vi "ProFile_Measure.vi"(1 "Ceiling":sgl=4.0, 2 "error in":errorcluster caption="Error In") -> (0 "error out":errorcluster caption="Error Out")   [LabVIEW 2016]
doc: "2D motor scan example Vi."
uses:
  Utility/Global Constants.vi
  Utility/Global_Array.vi
  Utility/Global_Stage.vi
panel:
  in  "Y-Axis Scanner align":sgl=0.15
  in  "X-Axis Scanner align":sgl=-0.64
  out "Value Handle":dbl[](array[numeric])
  out "Status?":bool
  out "RS":bool
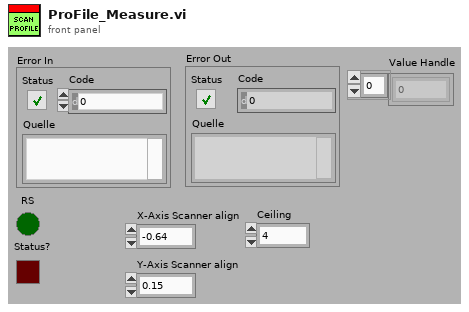
[diagram p1: front panel]
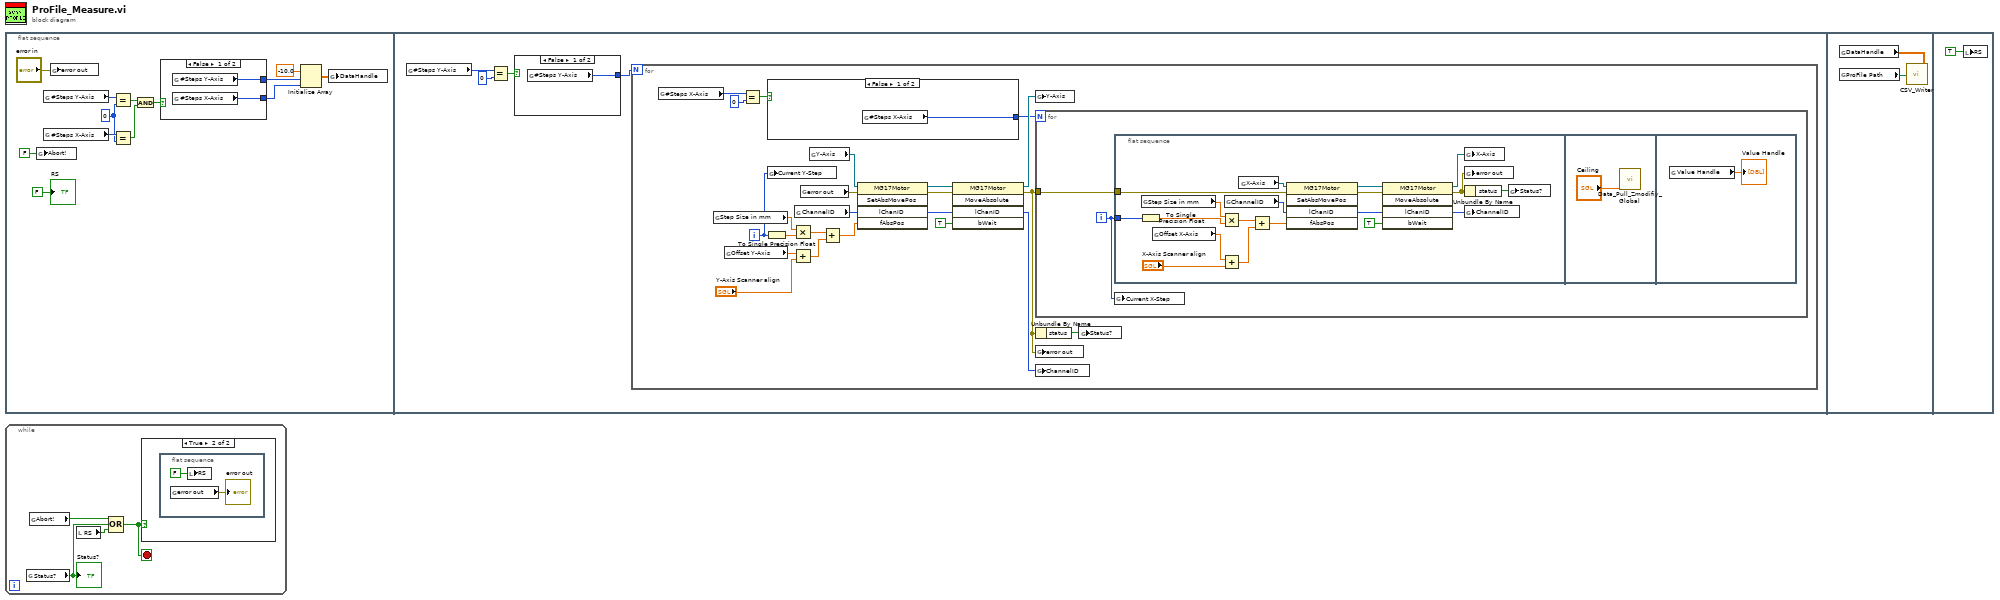
[diagram p0: block diagram]
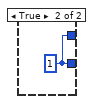
[diagram p3: hidden frame]
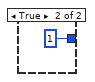
[diagram p4: hidden frame]
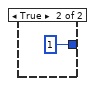
[diagram p5: hidden frame]
diagram:
  n1 = flat-sequence {
    frame #0 {
      w3 = 0 ("y")
      n2 = global write "Global Constants.vi" "Abort!"(FALSE) -> ()
      n3 = global read "Global Constants.vi" "#Steps Y-Axis"() -> (w8:i32)
      n4 = global read "Global Constants.vi" "#Steps X-Axis"() -> (w4:i32)
      n5 = global write "Global Constants.vi" "error out"("error in") -> ()
      n6 = Equal?(x=w8, y=w3) -> (x = y?=w7:bool)
      n7 = Equal?(x=w4, y=w3) -> (x = y?=w6:bool)
      n8 = And(x=w7, y=w6) -> (x .and. y?=w5:bool)
      n9 = case shown="False" w5 {
        tunnel: [w15 w16] -> w2
        tunnel: [w14 w16] -> w1
        frame False {
          n10 = global read "Global Constants.vi" "#Steps Y-Axis"() -> (w15:i32)
          n11 = global read "Global Constants.vi" "#Steps X-Axis"() -> (w14:i32)
        }
        frame True {
          w16 = 1
        }
      }
      n12 = Initialize Array(sgl -10.0 ("Element"), w2, w1) -> (w12:sgl[][])
      n13 = global write "Global_Array.vi" "DataHandle"(w12) -> ()
      "RS" <- FALSE ("Run Successful")
    }
    frame #1 {
      n14 = global read "Global Constants.vi" "#Steps Y-Axis"() -> (w20:i32)
      n15 = Equal?(x=w20, y=0) -> (x = y?=w19:bool)
      n16 = case shown="False" w19 {
        tunnel: [w21 1] -> w17
        frame False {
          n17 = global read "Global Constants.vi" "#Steps Y-Axis"() -> (w21:i32)
        }
        frame True {
        }
      }
      n18 = for {
        N: w17 -> [_]
        i -> [w30]
        n19 = global read "Global Constants.vi" "#Steps X-Axis"() -> (w25:i32)
        n20 = global read "Global Constants.vi" "Step Size in mm"() -> (w37:sgl)
        n21 = global read "Global Constants.vi" "Offset Y-Axis"() -> (w28:sgl)
        n22 = Equal?(x=w25, y=0) -> (x = y?=w24:bool)
        n23 = To Single Precision Float(number=w30) -> (single precision float=w42:sgl)
        n24 = case shown="False" w24 {
          tunnel: [w46 1 ("#Steps Y-Axis")] -> w26
          frame False {
            n25 = global read "Global Constants.vi" "#Steps X-Axis"() -> (w46:i32)
          }
          frame True {
          }
        }
        n26 = global write "Global Constants.vi" "Current Y-Step"(w30) -> ()
        n27 = Multiply(x=w37, y=w42) -> (x*y=w40:sgl)
        n28 = Add(x=w28, y="Y-Axis Scanner align") -> (x+y=w27:sgl)
        n29 = global read "Global_Stage.vi" "ChannelID"() -> (w35:i32)
        n30 = global read "Global Constants.vi" "error out"() -> (w31:errorcluster)
        n31 = global read "Global_Stage.vi" "Y-Axis"() -> (w36:refnum<k7>)
        n32 = Add(x=w40, y=w27) -> (x+y=w39:sgl)
        n33 = invoke class="MG17Motor" method="SetAbsMovePos"(reference=w36, error in=w31, "lChanID"=w35, "fAbsPos"=w39) -> (reference out=w41:refnum<k7>, error out=w45:errorcluster, "lChanID"=w43:i32)  [unwired: 1 in, 2 out]
        n34 = invoke class="MG17Motor" method="MoveAbsolute"(reference=w41, error in=w45, "lChanID"=w43, "bWait"=TRUE) -> (reference out=w33:refnum<k7>, error out=w32:errorcluster, "lChanID"=w34:i32)  [unwired: 1 in, 2 out]
        n35 = global write "Global_Stage.vi" "Y-Axis"(w33) -> ()
        n36 = for {
          N: w26 -> [_]
          tunnel: w32 -> [w49]
          i -> [w48]
          n37 = flat-sequence {
            tunnel: w48 -> [w63]
            tunnel: w49 -> [w53]
            frame #0 {
              n38 = To Single Precision Float(number=w63) -> (single precision float=w65:sgl)
              n39 = global read "Global Constants.vi" "Step Size in mm"() -> (w58:sgl)
              n40 = global read "Global Constants.vi" "Offset X-Axis"() -> (w52:sgl)
              n41 = Multiply(x=w58, y=w65) -> (x*y=w62:sgl)
              n42 = Add(x=w52, y="X-Axis Scanner align") -> (x+y=w50:sgl)
              n43 = global read "Global_Stage.vi" "ChannelID"() -> (w56:i32)
              n44 = global read "Global_Stage.vi" "X-Axis"() -> (w57:refnum<k7>)
              n45 = Add(x=w62, y=w50) -> (x+y=w61:sgl)
              n46 = invoke class="MG17Motor" method="SetAbsMovePos"(reference=w57, error in=w53, "lChanID"=w56, "fAbsPos"=w61) -> (reference out=w64:refnum<k7>, error out=w68:errorcluster, "lChanID"=w67:i32)  [unwired: 1 in, 2 out]
              n47 = invoke class="MG17Motor" method="MoveAbsolute"(reference=w64, error in=w68, "lChanID"=w67, "bWait"=TRUE) -> (reference out=w55:refnum<k7>, error out=w60:errorcluster, "lChanID"=w54:i32)  [unwired: 1 in, 2 out]
              n48 = global write "Global_Stage.vi" "X-Axis"(w55) -> ()
              n49 = global write "Global Constants.vi" "error out"(w60) -> ()
              n50 = Unbundle By Name(w60) -> ("status"=w59:bool)
              n51 = global write "Global_Stage.vi" "ChannelID"(w54) -> ()
              n52 = global write "Global Constants.vi" "Status?"(w59) -> ()
            }
            frame #1 {
              n53 = call "Data_Pull_Zmodifiy_Global.vi"("Ceiling"="Ceiling") -> ()
            }
            frame #2 {
              n54 = global read "Global_Array.vi" "Value Handle"() -> (→"Value Handle":dbl[])
            }
          }
          n55 = global write "Global Constants.vi" "Current X-Step"(w48) -> ()
        }
        n56 = Unbundle By Name(w32) -> ("status"=w38:bool)
        n57 = global write "Global Constants.vi" "error out"(w32) -> ()
        n58 = global write "Global_Stage.vi" "ChannelID"(w34) -> ()
        n59 = global write "Global Constants.vi" "Status?"(w38) -> ()
      }
    }
    frame #2 {
      n60 = global read "Global_Array.vi" "DataHandle"() -> (w72:sgl[][])
      n61 = global read "Global Constants.vi" "ProFile Path"() -> (w71:path)
      n62 = call "CSV_Writer.vi"("Array In"=w72, "ProFile In"=w71) -> ()
    }
    frame #3 {
      n63 = local write "RS"(TRUE) -> ()
    }
  }
  n64 = while {
    stop <- w76 stop-if-true
    n65 = global read "Global Constants.vi" "Status?"() -> (w75:bool)
    "Status?" <- w75
    n66 = global read "Global Constants.vi" "Abort!"() -> (w74:bool)
    n67 = local read "RS"() -> (w77:bool)
    n68 = Compound Arithmetic op=OR(w74, w75, w77) -> (w76:bool)
    n69 = case shown="True" w76 {
      frame False {
      }
      frame True {
        n70 = flat-sequence {
          frame #0 {
            n71 = global read "Global Constants.vi" "error out"() -> (→"error out":errorcluster)
            n72 = local write "RS"(FALSE) -> ()
          }
        }
      }
    }
  }
